vi "Build String Filter.vi"(8 "error in (no error)":errorcluster, 9 "Comparison Value":string, 10 "Comparison Method":T1(ring), 11 "String Filters in":refnum<class "String Filters.lvclass">) -> (0 "error out":errorcluster, 3 "String Filters out":refnum<class "String Filters.lvclass">)   [LabVIEW 2017, in "Assert API Components.lvlib" / "String Filters.lvclass"]
uses:
  String Filters.lvclass
  String Filters.lvclass/String Filters.ctl
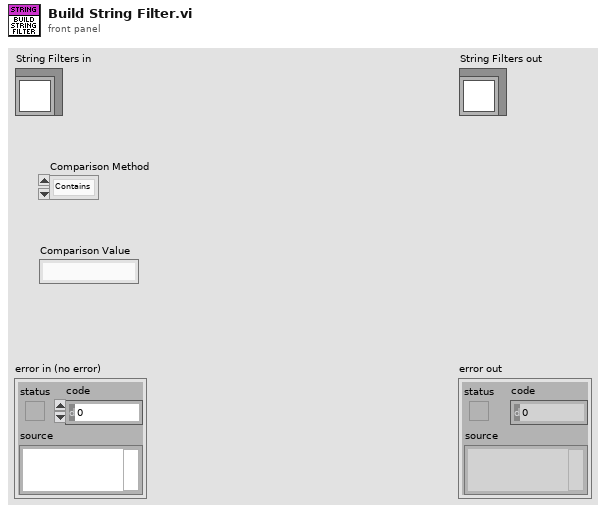
[diagram p1: front panel]
types:
  T1 = enum16{"Contains", "Does Not Contain", "Starts With", "Equals", "Does Not Equal"}
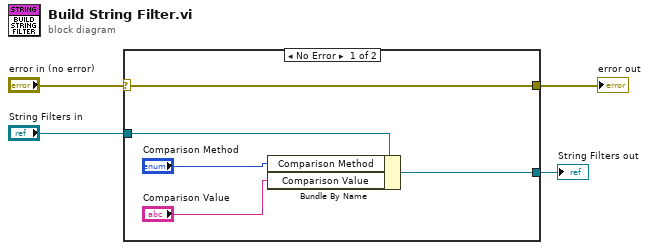
[diagram p0: block diagram]
diagram:
  n1 = case shown="No Error" "error in (no error)" {
    selector: "error in (no error)" -> [w8 w11]
    tunnel: [w8 w11] -> w3
    tunnel: [w7 w10] -> w1
    tunnel: "String Filters in" -> [w9 w10]
    frame No Error {
      n2 = Bundle By Name(cluster=w9, "Comparison Method"="Comparison Method", "Comparison Value"="Comparison Value") -> (w7:refnum<class "String Filters.lvclass">)
    }
    frame Error {
    }
  }
  "error out" <- w3
  "String Filters out" <- w1
